vi "OldClimbNetworkingGlobal.vi"() -> ()   [LabVIEW 2023]
panel:
  out "RevLimLeft":bool
  out "FowardLimitSwitchLeft":bool
  out "RevLimRight":bool
  out "OnTargetLeft":bool
  out "FowardLimitSwitchRight":bool
  out "OnTargetRight":bool
  in  "SensorPosLeft":dbl
  in  "MotorOutRight":dbl
  in  "Demand":dbl
  in  "SensorPosRight":dbl
  in  "MotorOutLeft":dbl
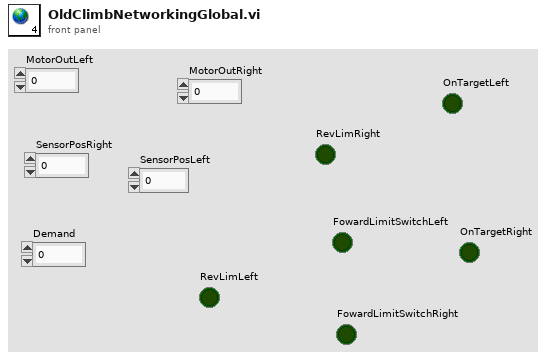
[diagram p1: front panel]
diagram:
